vi "Configure Modulation Source.vi"(0 "VISA resource name":refnum<visa-resource-name>, 1 "Internal Waveform (0: Sine)":u16(ring) items=["Sine", "Triangle", "Square", "Ramp", "Noise", "Dual-Sine", "Swept-Sine"], 2 "Modulation Path (1)":u16(ring)=1 items=["1"=1, "2"=2], 3 "Modulation Type (0: Amplitude Modulation)":u16(ring) items=["Amplitude Modulation", "Frequency Modulation", "Phase Modulation"], 5 "Modulation Source (0: Internal1)":u16(ring) items=["Internal1", "Internal2", "External1", "External2", "Sweep", "Dual", "Noise1", "Noise2"], 7 "Internal Frequency (400 Hz)":dbl=400.0, 9 "Alternate Internal Frequency (400 Hz)":dbl=400.0, 11 "error in (no error)":errorcluster, 12 "External Coupling (1: DC)":u16(ring)=1 items=["AC", "DC"], 13 "External Impedance (0: 50 Ohms)":u16(ring) items=["50 Ohms", "600 Ohms"]) -> (4 "VISA resource name out":refnum<visa-resource-name>, 15 "error out":errorcluster)   [LabVIEW 2018, in "Agilent PSG MXG Series.lvlib"]
doc: "Configures the modulation source and relative parameters of a specific modulation.\n\n<B>Notes:</B>\n(1) This VI is <B>NOT</B> valid in E8247C.\n\n(2) For E8257D, E8267D, N5161A, N5162A, N5181A, N5182A, N5183A, N5171B, N5172B, N5181B, N5182B, N5173B, N5183B, this VI is valid only when the instrument installs <B>Option UNT</B> (AM, FM, phase modulation).\n\n(3) For N5171B, N5172B, N5181B, N5182B, N5173B, N5183B, only Modulation Type, Modulation Path and Modulation Source are valid."
uses:
  Agilent PSG MXG Series.lvlib
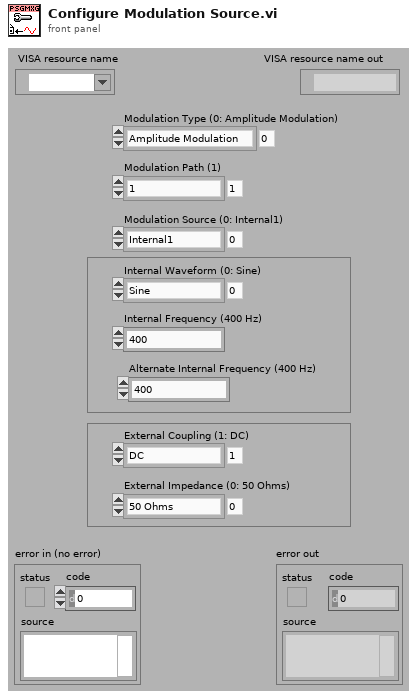
[diagram p1: front panel]
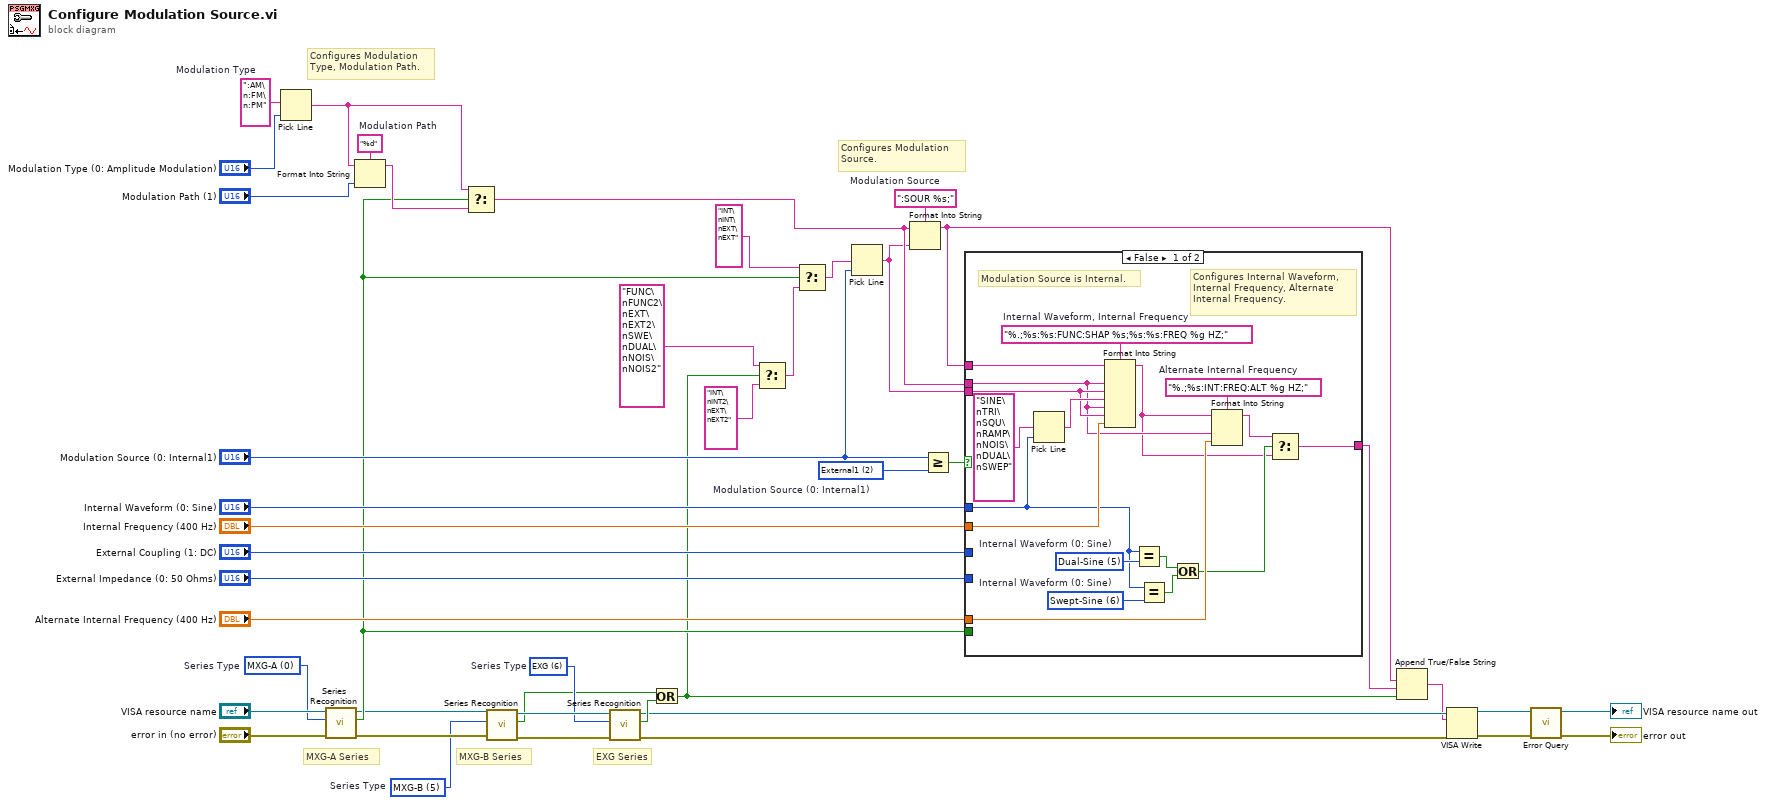
[diagram p0: block diagram]
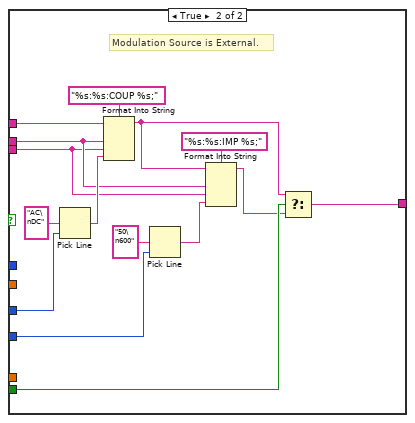
[diagram p2: hidden frame]
diagram:
  w12 = u16 6 items=["MXG-A", "PSG", "PSG-A", "PSG-C", "PSG-D", "MXG-B", "EXG"]  # Series Type
  w15 = u16 5 items=["MXG-A", "PSG", "PSG-A", "PSG-C", "PSG-D", "MXG-B", "EXG"]  # Series Type
  w18 = u16 0 items=["MXG-A", "PSG", "PSG-A", "PSG-C", "PSG-D", "MXG-B", "EXG"]  # Series Type
  w37 = u16 2 items=["Internal1", "Internal2", "External1", "External2"]  # Modulation Source (0: Internal1)
  w38 = ":SOUR %s;"  # Modulation Source
  w41 = "%d"  # Modulation Path
  w44 = ":AM\n:FM\n:PM"  # Modulation Type
  # "EXG Series"
  # "MXG-B Series"
  # "Configures Modulation\nSource."
  # "Configures Modulation\nType, Modulation Path."
  # "MXG-A Series"
  n1 = Pick Line(multi-line string=w44, line index="Modulation Type (0: Amplitude Modulation)") -> (output string=w40:string)  [unwired: 1 out]
  n2 = call "Series Recognition.vi"("error in (no error)"="error in (no error)", "Series Type (0: MXG)"=w18, "VISA resource name"="VISA resource name") -> ("error out"=w16:errorcluster, "Is Series Correct"=w23:bool, "VISA resource name out"=w17:refnum<visa-resource-name>)  [unwired: 6 out]
  n3 = Format Into String(format string=w41, initial string=w40, "Modulation Path (1)") -> (resulting string=w39:string)  [unwired: 1 in, 1 out]
  n4 = Select(t=w40, s=w23, f=w39) -> (s? t:f=w34:string)
  n5 = call "Series Recognition.vi"("error in (no error)"=w16, "Series Type (0: MXG)"=w15, "VISA resource name"=w17) -> ("error out"=w13:errorcluster, "Is Series Correct"=w10:bool, "VISA resource name out"=w14:refnum<visa-resource-name>)  [unwired: 6 out]
  n6 = call "Series Recognition.vi"("error in (no error)"=w13, "Series Type (0: MXG)"=w12, "VISA resource name"=w14) -> ("error out"=w6:errorcluster, "Is Series Correct"=w11:bool, "VISA resource name out"=w5:refnum<visa-resource-name>)  [unwired: 6 out]
  n7 = Or(x=w10, y=w11) -> (x .or. y?=w3:bool)
  n8 = Select(t="FUNC\nFUNC2\nEXT\nEXT2\nSWE\nDUAL\nNOIS\nNOIS2" ("multi-line string"), s=w3, f="INT\nINT2\nEXT\nEXT2" ("multi-line string")) -> (s? t:f=w7:string)
  n9 = Select(t="INT\nINT\nEXT\nEXT" ("multi-line string"), s=w23, f=w7) -> (s? t:f=w29:string)
  n10 = Pick Line(multi-line string=w29, line index="Modulation Source (0: Internal1)") -> (output string=w33:string)  [unwired: 1 out]
  n11 = Format Into String(format string=w38, initial string=w34, w33) -> (resulting string=w1:string)  [unwired: 1 in, 1 out]
  n12 = Greater Or Equal?(x="Modulation Source (0: Internal1)", y=w37) -> (x >= y?=w35:bool)
  n13 = case shown="False" w35 {
    tunnel: w34 -> [w56 w72]
    tunnel: w33 -> [w59 w71]
    tunnel: "Internal Waveform (0: Sine)" -> [w53 _]
    tunnel: "Internal Frequency (400 Hz)" -> [w58 _]
    tunnel: "External Coupling (1: DC)" -> [_ w74]
    tunnel: "External Impedance (0: 50 Ohms)" -> [_ w68]
    tunnel: w23 -> [_ w67]
    tunnel: [w46 w64] -> w2
    tunnel: "Alternate Internal Frequency (400 Hz)" -> [w55 _]
    tunnel: w1 -> [w45 w63]
    frame False {
      w52 = u16 6 items=["Sine", "Triangle", "Square", "Ramp", "Noise", "Dual-Sine", "Swept-Sine"]  # Internal Waveform (0: Sine)
      w57 = "%.;%s:INT:FREQ:ALT %g HZ;"  # Alternate Internal Frequency
      w54 = u16 5 items=["Sine", "Triangle", "Square", "Ramp", "Noise", "Dual-Sine", "Swept-Sine"]  # Internal Waveform (0: Sine)
      w62 = "%.;%s:%s:FUNC:SHAP %s;%s:%s:FREQ %g HZ;"  # Internal Waveform, Internal Frequency
      # "Configures Internal Waveform,\nInternal Frequency, Alternate\nInternal Frequency."
      # "Modulation Source is Internal."
      n14 = Pick Line(multi-line string="SINE\nTRI\nSQU\nRAMP\nNOIS\nDUAL\nSWEP", line index=w53) -> (output string=w61:string)  [unwired: 1 out]
      n15 = Format Into String(format string=w62, initial string=w45, w56, w59, w61, w56, w59, w58) -> (resulting string=w47:string)  [unwired: 1 in, 1 out]
      n16 = Equal?(x=w53, y=w54) -> (x = y?=w51:bool)
      n17 = Equal?(x=w53, y=w52) -> (x = y?=w50:bool)
      n18 = Or(x=w51, y=w50) -> (x .or. y?=w49:bool)
      n19 = Format Into String(format string=w57, initial string=w47, w56, w55) -> (resulting string=w48:string)  [unwired: 1 in, 1 out]
      n20 = Select(t=w48, s=w49, f=w47) -> (s? t:f=w46:string)
    }
    frame True {
      # "Modulation Source is External."
      n21 = Pick Line(multi-line string="AC\nDC", line index=w74) -> (output string=w76:string)  [unwired: 1 out]
      n22 = Format Into String(format string="%s:%s:COUP %s;", initial string=w63, w72, w71, w76) -> (resulting string=w66:string)  [unwired: 1 in, 1 out]
      n23 = Pick Line(multi-line string="50\n600", line index=w68) -> (output string=w70:string)  [unwired: 1 out]
      n24 = Format Into String(format string="%s:%s:IMP %s;", initial string=w66, w72, w71, w70) -> (resulting string=w65:string)  [unwired: 1 in, 1 out]
      n25 = Select(t=w66, s=w67, f=w65) -> (s? t:f=w64:string)
    }
  }
  n26 = Append True/False String(1:w3, 2:w2, 3:w1) -> (0:w4:string)  [unwired: 1 out]
  n27 = VISA Write(VISA resource name=w5, write buffer=w4, error in (no error)=w6) -> (VISA resource name out=w26:refnum<visa-resource-name>, error out=w25:errorcluster)  [unwired: 1 out]
  n28 = call "Error Query.vi"("error in (no error)"=w25, "VISA resource name"=w26) -> ("error out"=→"error out":errorcluster, "VISA resource name out"=→"VISA resource name out":refnum<visa-resource-name>)  [unwired: 8 out]
